vi "Clear Dictionaries.vi"(11 "error in (no error)":errorcluster) -> (15 "error out":errorcluster)   [LabVIEW 2023, in "RFCalAndFixtureCharact.Common.lvlib"]
uses:
  RFCalAndFixtureCharact.Common.lvlib
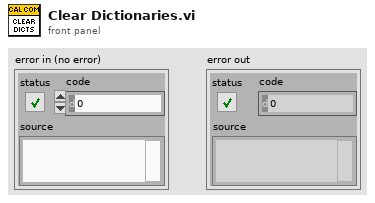
[diagram p1: front panel]
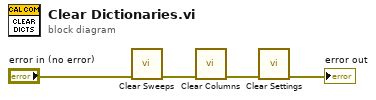
[diagram p0: block diagram]
diagram:
  n1 = call "Clear Sweeps.vi"("error in (no error)"="error in (no error)") -> ("error out"=w3:errorcluster)  [unwired: 14 in]
  n2 = call "Clear Columns.vi"("error in (no error)"=w3) -> ("error out"=w2:errorcluster)  [unwired: 14 in]
  n3 = call "Clear Settings.vi"("error in (no error)"=w2) -> ("error out"=→"error out":errorcluster)  [unwired: 14 in]
